vi "Set_gain.vi"(8 "error in":errorcluster, 11 "Gain":u8 format="%02x") -> (0 "error out":errorcluster)   [LabVIEW 2018]
panel:
  # "Gain\n00: 1x\n01: 4x\n10: 16x\n11: 60x"
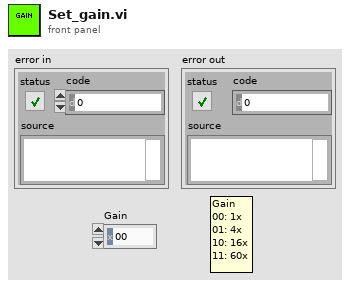
[diagram p1: front panel]
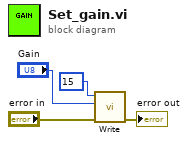
[diagram p0: block diagram]
diagram:
  n1 = call "Write.vi"("error in"="error in", "Data to write"="Gain", "Address"=u8 15 ("Slave Address (7-bit)")) -> ("error out"=→"error out":errorcluster)  [unwired: 8 in]
